vi "POP_GOOGLE.vi"(8 "error in":errorcluster, 11 "chemin":path) -> (0 "error out":errorcluster caption="sortie d'erreur", 3 "standard output":string caption="sortie standard")   [LabVIEW 2020]
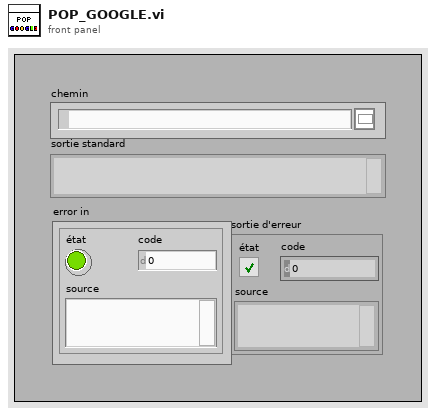
[diagram p1: front panel]
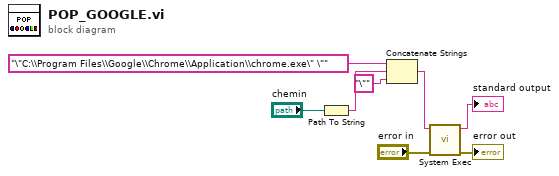
[diagram p0: block diagram]
diagram:
  n1 = Path To String(path="chemin") -> (string=w2:string)
  n2 = Concatenate Strings("\"C:\\Program Files\\Google\\Chrome\\Application\\chrome.exe\" \"", w2, "\"" ("chaîne")) -> (w6:string)
  n3 = call <vilib>:"System Exec.vi"("error in (no error)"="error in", "command line"=w6) -> ("error out"=→"error out":errorcluster, "standard output"=→"standard output":string)  [unwired: 6 in, 2 out]
